vi "Grabber Position to Angles.vi"(8 "Forearm Length":dbl, 9 "Backarm Length":dbl, 10 "Y Initial":dbl, 11 "X Initial":dbl) -> (0 "Forearm Angle\nDegrees 2":dbl format="%.2f", 1 "Backarm Angle\nDegrees 2":dbl format="%.2f", 2 "Forearm Angle\nDegrees 1":dbl format="%.2f", 3 "Backarm Angle\nDegrees 1":dbl format="%.2f")   [LabVIEW 2017]
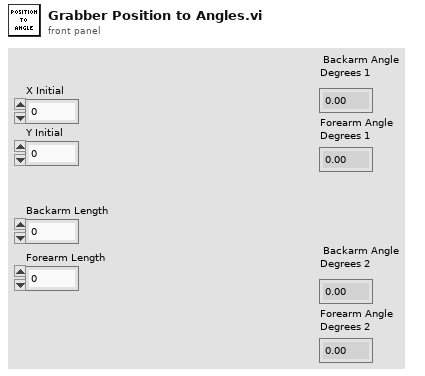
[diagram p1: front panel]
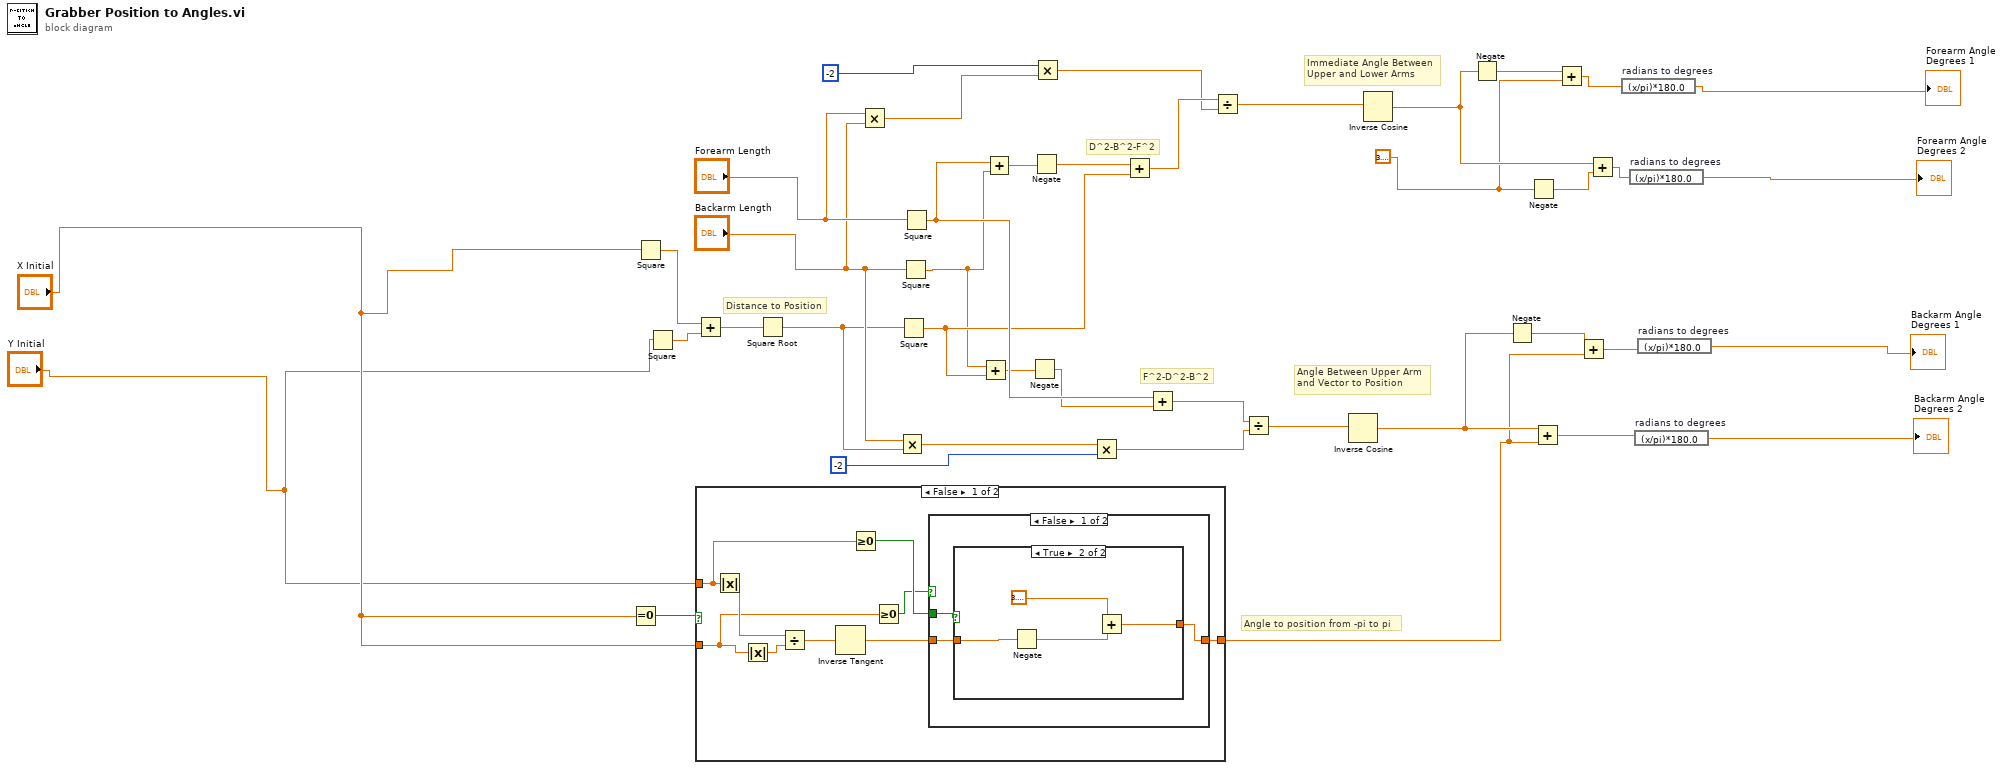
[diagram p0: block diagram]
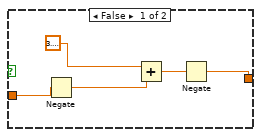
[diagram p2: hidden frame]
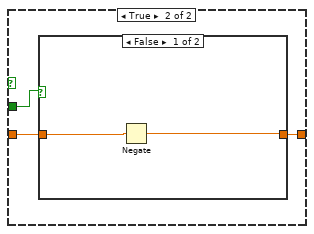
[diagram p3: hidden frame]
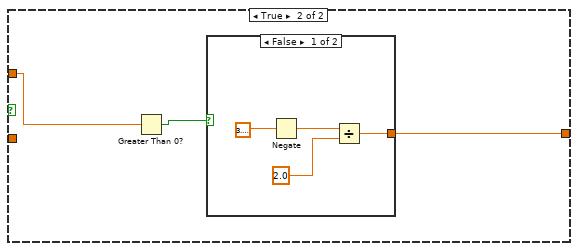
[diagram p5: hidden frame]
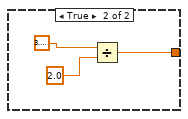
[diagram p6: hidden frame]
diagram:
  w16 = 3.141592653589793
  # "Angle Between Upper Arm\nand Vector to Position"
  # "Immediate Angle Between\nUpper and Lower Arms"
  # "F^2-D^2-B^2"
  # "D^2-B^2-F^2"
  # "Distance to Position"
  # "Angle to position from -pi to pi"
  n1 = Equal To 0?(x="X Initial") -> (x = 0?=w7:bool)
  n2 = Square(x="X Initial") -> (x^2=w41:dbl)
  n3 = Square(x="Y Initial") -> (x^2=w40:dbl)
  n4 = case shown="False" w7 {
    tunnel: "Y Initial" -> [w46 w70]
    tunnel: [w44 w69] -> w8
    tunnel: "X Initial" -> [w45 _]
    frame False {
      n5 = Absolute Value(x=w46) -> (abs(x)=w47:dbl)
      n6 = Absolute Value(x=w45) -> (abs(x)=w48:dbl)
      n7 = Divide(x=w47, y=w48) -> (x/y=w49:dbl)
      n8 = Inverse Tangent(1:w49) -> (0:w50:dbl)
      n9 = Greater Or Equal To 0?(x=w46) -> (x >= 0?=w43:bool)
      n10 = Greater Or Equal To 0?(x=w45) -> (x >= 0?=w42:bool)
      n11 = case shown="False" w42 {
        tunnel: w43 -> [w53 w65]
        tunnel: w50 -> [w52 w64]
        tunnel: [w51 w63] -> w44
        frame False {
          n12 = case shown="True" w53 {
            tunnel: w52 -> [w56 w62]
            tunnel: [w54 w59] -> w51
            frame False {
              n13 = Negate(x=w56) -> (-x=w58:dbl)
              n14 = Add(x=3.141592653589793, y=w58) -> (x+y=w55:dbl)
              n15 = Negate(x=w55) -> (-x=w54:dbl)
            }
            frame True {
              n16 = Negate(x=w62) -> (-x=w60:dbl)
              n17 = Add(x=3.141592653589793, y=w60) -> (x+y=w59:dbl)
            }
          }
        }
        frame True {
          n18 = case shown="False" w65 {
            tunnel: w64 -> [w67 w68]
            tunnel: [w66 w68] -> w63
            frame False {
              n19 = Negate(x=w67) -> (-x=w66:dbl)
            }
            frame True {
            }
          }
        }
      }
    }
    frame True {
      n20 = Greater Than 0?(x=w70) -> (x > 0?=w71:bool)
      n21 = case shown="False" w71 {
        tunnel: [w73 w78] -> w69
        frame False {
          n22 = Negate(x=3.141592653589793) -> (-x=w74:dbl)
          n23 = Divide(x=w74, y=2.0) -> (x/y=w73:dbl)
        }
        frame True {
          n24 = Divide(x=3.141592653589793, y=2.0) -> (x/y=w78:dbl)
        }
      }
    }
  }
  n25 = Add(x=w41, y=w40) -> (x+y=w39:dbl)
  n26 = Square Root(x=w39) -> (sqrt(x)=w36:dbl)
  n27 = Multiply(x="Forearm Length", y="Backarm Length") -> (x*y=w35:dbl)
  n28 = Multiply(x="Backarm Length", y=w36) -> (x*y=w32:dbl)
  n29 = Square(x=w36) -> (x^2=w28:dbl)
  n30 = Square(x="Backarm Length") -> (x^2=w27:dbl)
  n31 = Square(x="Forearm Length") -> (x^2=w29:dbl)
  n32 = Add(x=w27, y=w28) -> (x+y=w25:dbl)
  n33 = Add(x=w29, y=w27) -> (x+y=w31:dbl)
  n34 = Negate(x=w25) -> (-x=w26:dbl)
  n35 = Negate(x=w31) -> (-x=w30:dbl)
  n36 = Multiply(x=-2, y=w35) -> (x*y=w23:dbl)
  n37 = Multiply(x=w32, y=-2) -> (x*y=w21:dbl)
  n38 = Add(x=w30, y=w28) -> (x+y=w24:dbl)
  n39 = Add(x=w29, y=w26) -> (x+y=w22:dbl)
  n40 = Divide(x=w24, y=w23) -> (x/y=w20:dbl)
  n41 = Divide(x=w22, y=w21) -> (x/y=w19:dbl)
  n42 = Inverse Cosine(1:w19) -> (0:w10:dbl)
  n43 = Inverse Cosine(1:w20) -> (0:w18:dbl)
  n44 = Negate(x=w18) -> (-x=w17:dbl)
  n45 = Negate(x=w10) -> (-x=w9:dbl)
  n46 = Negate(x=w16) -> (-x=w15:dbl)
  n47 = Add(x=w10, y=w8) -> (x+y=w11:dbl)
  n48 = Add(x=w17, y=w16) -> (x+y=w14:dbl)
  n49 = Add(x=w9, y=w8) -> (x+y=w12:dbl)
  n50 = Add(x=w18, y=w15) -> (x+y=w13:dbl)
  n51 = expression code="(x/pi)*180.0" "radians to degrees"(w14) -> (→"Forearm Angle\nDegrees 1":dbl)
  n52 = expression code="(x/pi)*180.0" "radians to degrees"(w13) -> (→"Forearm Angle\nDegrees 2":dbl)
  n53 = expression code="(x/pi)*180.0" "radians to degrees"(w11) -> (→"Backarm Angle\nDegrees 2":dbl)
  n54 = expression code="(x/pi)*180.0" "radians to degrees"(w12) -> (→"Backarm Angle\nDegrees 1":dbl)
